vi "Read TestManager.vi"(11 "Properties in":refnum<class "Properties.lvclass">) -> (2 "Test Manager":refnum<class "Basic Test Manager.lvclass">, 3 "Properties out":refnum<class "Properties.lvclass">)   [LabVIEW 2020, in "Caraya.lvlib" / "Properties.lvclass"]
uses:
  Properties.lvclass
  Basic Test Manager/Basic Test Manager.lvclass
  Properties.lvclass/Properties.ctl
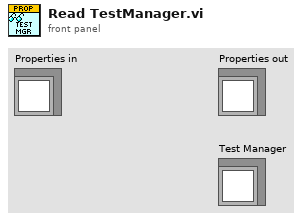
[diagram p1: front panel]
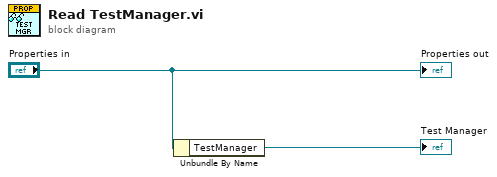
[diagram p0: block diagram]
diagram:
  n1 = Unbundle By Name("Properties in") -> ("TestManager"=→"Test Manager":refnum<class "Basic Test Manager.lvclass">)
  "Properties out" <- "Properties in"
